vi "Slider Get Offset.vi"(9 "Index":i32, 10 "LBCB Number":T1, 11 "DofType":T2) -> (2 "Offset":dbl)   [LabVIEW 2009]
uses:
  Data Access Objects/Limits/DofTypes.ctl
  Data Access Objects/Metadata/LBCB Number.ctl
  Global Data/Transactions/Dataset Type.ctl
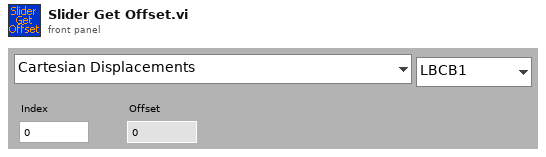
[diagram p1: front panel]
types:
  T1 = typedef "LBCB Number.ctl" = enum16{"LBCB1", "LBCB2"}
  T2 = typedef "DofTypes.ctl" = enum16{"Cartesian Displacements", "Cartesian Forces & Moments", "Actuator Displacements", "Actuator Forces", "Cartesian Increments", "Actuator Increments"}
  T3 = typedef "Dataset Type.ctl" = enum16{"LVDT", "Load Cell", "Actuator Command", "Servo Error", "Displacement Command", "Displacement", "Force"}
  T4 = typedef "Dataset Source.ctl" = enum16{"LBCB 1", "LBCB 2", "Combined", "External Sensors"}
  T5 = typedef "Dataset Transaction Id.ctl" = cluster{"Dataset Source":T4, "Dataset Type":T3, "Hold":T6, "Volts":T6, "Tag":string}
  T6 = typedef "Yes No Button.ctl" = bool
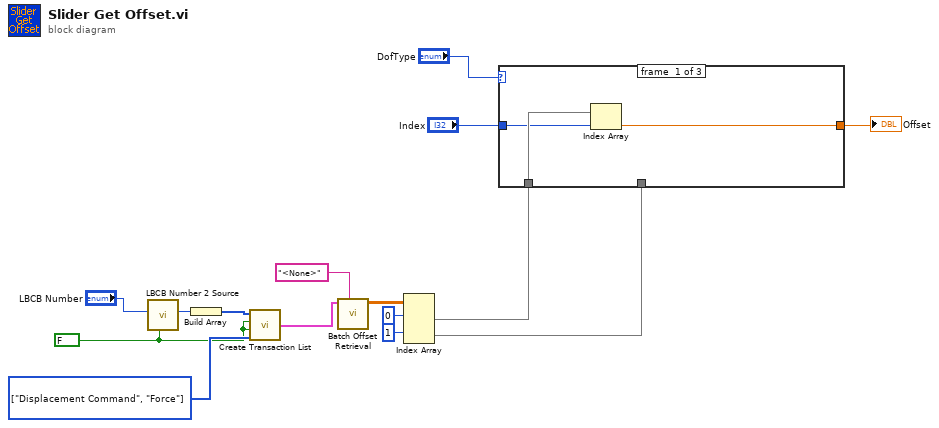
[diagram p0: block diagram]
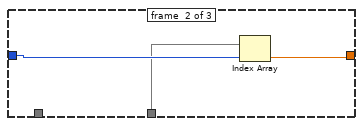
[diagram p2: hidden frame]
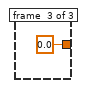
[diagram p3: hidden frame]
diagram:
  w9 = T3[] [enum."Displacement Command", enum."Force"] items=["LVDT", "Load Cell", "Actuator Command", "Servo Error", "Displacement Command", "Displacement", "Force"] ("Types")
  w1 = FALSE ("Volts")
  n1 = call "LBCB Number 2 Source.vi"("Combined"=w1, "LBCB Number"="LBCB Number") -> ("Dataset Source"=w11:T4)  [unwired: 9 in]
  n2 = Build Array(w11) -> (w10:T4[])
  n3 = call "Create Transaction List.vi"("Types"=w9, "Hold"=w1, "Volts"=w1, "Sources"=w10) -> ("Transactions"=w8:T5[])
  n4 = call "Batch Offset Retrieval.vi"("Tag"="<None>", "Transactions"=w8) -> ("Data"=w6:dbl[][])  [unwired: 8 in, 1 out]
  n5 = Index Array(array=w6, index (row) #1=0 ("index (row)"), index (row) #2=1 ("index (row)")) -> (element #1=w3:dbl[], element #2=w2:dbl[])  [unwired: 2 in]
  n6 = case shown="\"Cartesian Forces & Moments\"" "DofType" {
    tunnel: w3 -> [w18 _ _]
    tunnel: w2 -> [_ w19 _]
    tunnel: "Index" -> [w17 w21 _]
    tunnel: [w16 w20 0.0 ("Numeric")] -> w13
    frame #0 {
      n7 = Index Array(array=w18, index=w17) -> (element=w16:dbl)
    }
    frame #1 {
      n8 = Index Array(array=w19, index=w21) -> (element=w20:dbl)
    }
    frame #2 {
    }
  }
  "Offset" <- w13
